vi "Read_Global_ini.vi"(8 "Error In":errorcluster, 11 "Global ini path":path) -> (0 "Error Out":errorcluster, 1 "Session id name":string, 2 "Global Cluster":T1)   [LabVIEW 2017]
doc: "This subVI fetches all the parameters from the global ini file and parameters are relevant to test case.\n\n<B>Path:</B>\n\\\\UltraSonic_Test_Scripts\\\\BF_INT_TESTSUITE_AUTO\\\\testcasename\\\\testcasename.ini\n\n<B>For Ex:</B>"
uses:
  <vilib>/Utility/config.llb/Read Key (String).vi
  <vilib>/Utility/config.llb/NI_LVConfig.lvlib
panel:
  out "Keys in ini":string[](array[string])
  # "READ FROM GLOBAL INI FILE"
  # "ERROR"
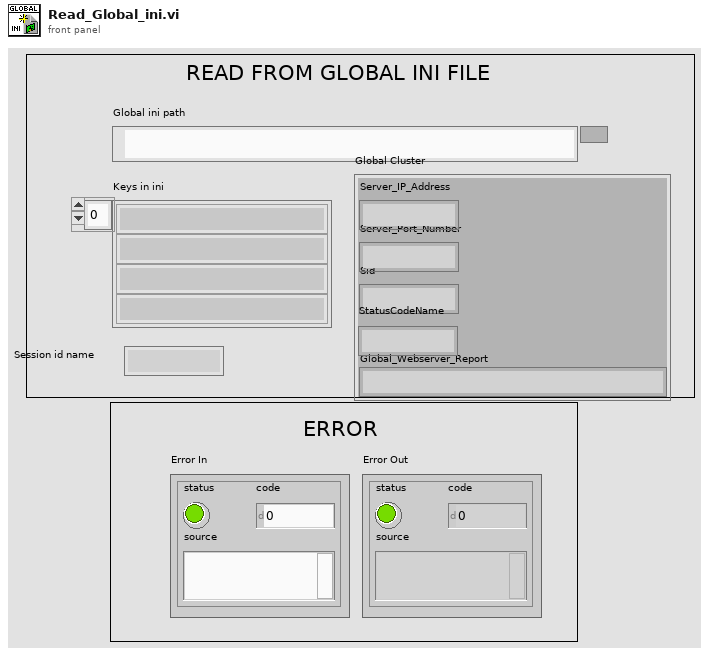
[diagram p1: front panel]
types:
  T1 = cluster{"Server_IP_Address":string, "Server_Port_Number":string, "Sid":string, "StatusCodeName":string, "Global_Webserver_Report":string}
  T2 = typedef "NI_LVConfig.lvlib/Config Data RefNum.ctl" = refnum<k1>
  T3 = cluster{"[0]":string, "[1]":string, "[2]":string, "[3]":string, "[4]":string}
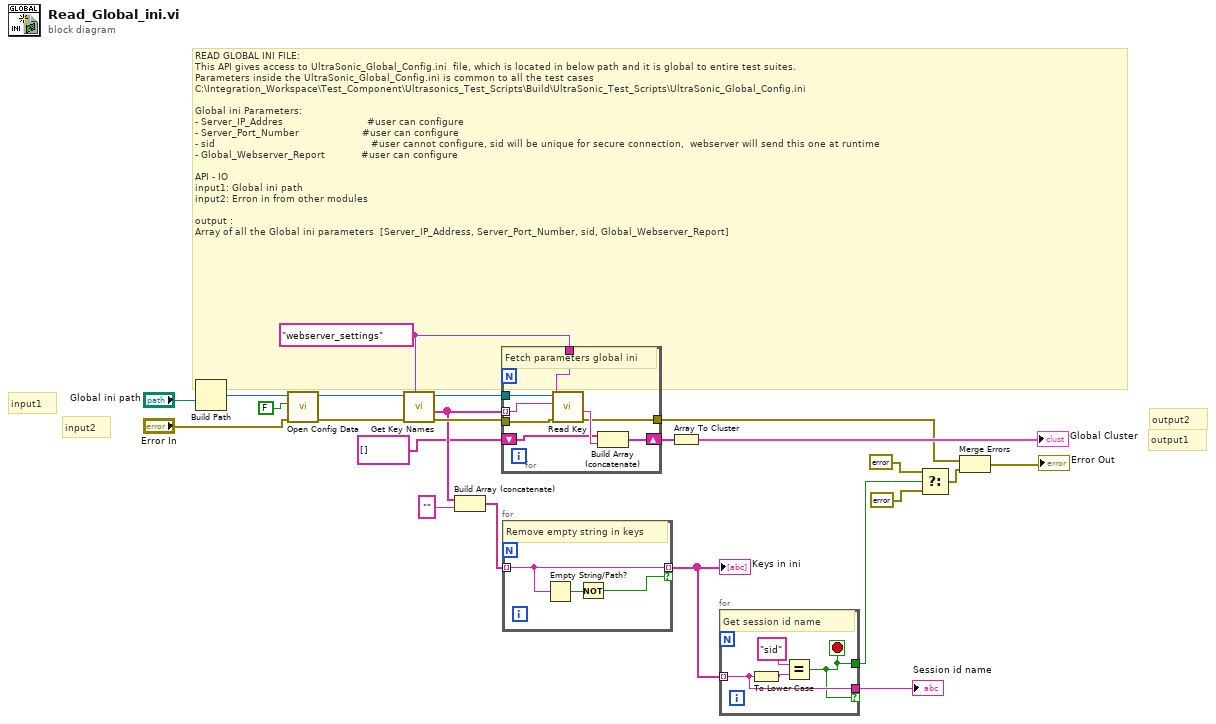
[diagram p0: block diagram]
diagram:
  w13 = "webserver_settings"
  # "output2"
  # "output1"
  # "input2"
  # "input1"
  # "READ GLOBAL INI FILE:\nThis API gives access to UltraSonic_Global_Config.ini  file, which is located in below path and it is global to entire test suites.\nParameters inside the UltraSonic_Global_Config.ini is common to all the test cases\nC:\\Integration_Workspace\\Test_Component\\Ultrasonics_Test_Scripts\\Build\\UltraSonic_Test_Scripts\\UltraSonic_Global_Config.ini \n\nGlobal ini Parameters:\n- Server_IP_Addres                            #user can configure\n- Server_Port_Number                     #user can configure\n- sid                                                    #user cannot configure, sid will be unique for secure connection,  webserver will send this one at runtime\n- Global_Webserver_Report            #user can configure\n\nAPI - IO\ninput1: Global ini path\ninput2: Erron in from other modules\n\noutput : \nArray of all the Global ini parameters  [Server_IP_Address, Server_Port_Number, sid, Global_Webserver_Report]"
  n1 = Build Path(name or relative path="Global ini path") -> (appended path=w22:path)  [unwired: 1 in]
  n2 = call <vilib>:"Open Config Data.vi"("error in (no error)"="Error In", "create file if necessary (T)"=FALSE ("create file if necessary? (T)"), "configuration file path"=w22) -> ("error out"=w20:errorcluster, "refnum"=w10:T2)  [unwired: 6 in, 1 out]
  n3 = call <vilib>:"Get Key Names.vi"("section"=w13, "error in (no error)"=w20, "refnum"=w10) -> ("error out"=w15:errorcluster, "key names"=w14:string[], "refnum out"=w16:T2)  [unwired: 5 in, 1 out]
  n4 = Build Array (concatenate)(w14, "") -> (w18:string[])
  n5 = for {
    tunnel: w14 -> [w29] mode=indexing
    tunnel: w16 -> [w31]
    tunnel: w15 -> [w30]
    tunnel: [w27] -> w4
    tunnel: w13 -> [w26]
    shift-right: [w25] -> w12
    shift-left: string[] [] -> [w24]
    # "Fetch parameters global ini"
    n6 = call-poly <vilib>:"Read Key.vi"("section"=w26, "error in (no error)"=w30, "key"=w29, "refnum"=w31) -> ("error out"=w27:errorcluster, "value"=w28:string)  [unwired: 2 in, 4 out]
    n7 = Build Array (concatenate)(w24, w28) -> (w25:string[])
  }
  n8 = for {
    tunnel: w18 -> [w33] mode=indexing
    tunnel: [w33] -> w8 mode=indexing if=w32
    # "Remove empty string in keys"
    n9 = Empty String/Path?(string/path=w33) -> (empty?=w34:bool)
    n10 = Not(x=w34) -> (.not. x?=w32:bool)
  }
  "Keys in ini" <- w8
  n11 = Array To Cluster(array=w12) -> (cluster=→"Global Cluster":T3)
  n12 = for {
    tunnel: w8 -> [w36] mode=indexing
    tunnel: [w36] -> w7 if=w35
    tunnel: [w35] -> w6
    stop <- w35 stop-if-true
    # "Get session id name"
    n13 = To Lower Case(string=w36) -> (all lower case string=w37:string)
    n14 = Equal?(x="sid", y=w37) -> (x = y?=w35:bool)
  }
  "Session id name" <- w7
  n15 = Select(t=errorcluster {"status"=FALSE, "code"=0, "source"=""} ("error constant"), s=w6, f=errorcluster {"status"=TRUE, "code"=0, "source"="Sid name is missing"} ("error constant")) -> (s? t:f=w5:errorcluster)
  n16 = Merge Errors(w4, w5) -> (→"Error Out":errorcluster)
